vi "Error Library.vi"(0 "Path":path, 2 "action":T2=enum."Register", 7 "Priority":bool, 11 "error in":errorcluster) -> (4 "Entry":T1, 8 "found?":bool, 15 "error thru":errorcluster)   [LabVIEW 2020]
uses:
  Error-Library Action.ctl
  Error Description.ctl
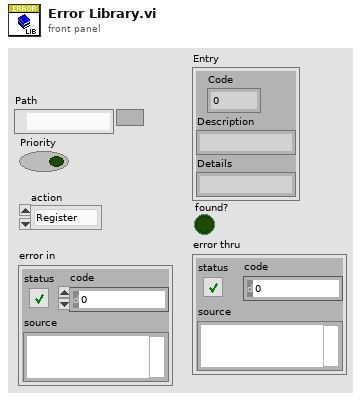
[diagram p1: front panel]
types:
  T1 = typedef "Error Description.ctl" = cluster{"Code":i32, "Description":string, "Details":string}
  T2 = typedef "Error-Library Action.ctl" = enum16{"NONE", "Register", "Read"}
  T3 = cluster{"code":i32, "source":string, "source":string}
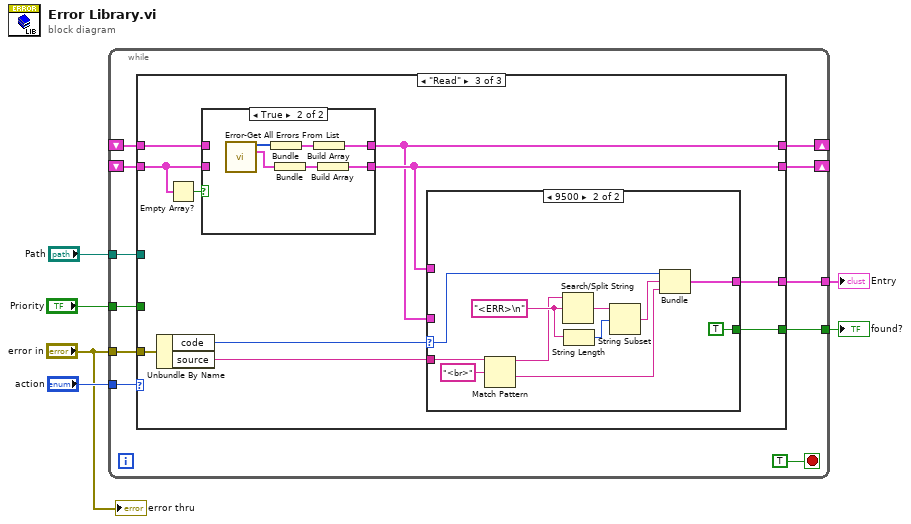
[diagram p0: block diagram]
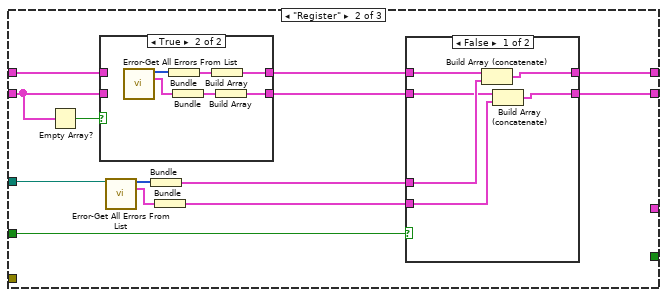
[diagram p3: hidden frame]
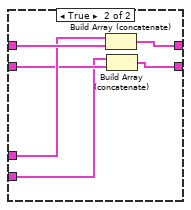
[diagram p4: hidden frame]
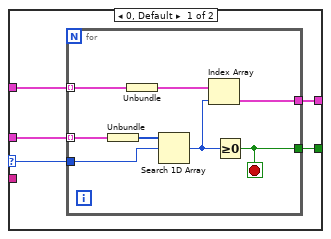
[diagram p6: hidden frame]
diagram:
  n1 = while {
    tunnel: "Path" -> [w16]
    tunnel: "Priority" -> [w15]
    tunnel: "action" -> [w14]
    shift-right: [w13] -> _
    shift-left: _ -> [w12]
    shift-right: [w11] -> _
    shift-left: _ -> [w10]
    tunnel: "error in" -> [w9]
    tunnel: [w8] -> w2
    tunnel: [w7] -> w1
    stop <- TRUE stop-if-true
    n2 = case shown="\"Read\"" w14 {
      tunnel: w16 -> [_ w27 _]
      tunnel: w15 -> [_ w22 _]
      tunnel: [w18 w23 w55] -> w13
      tunnel: w12 -> [w18 w30 w56]
      tunnel: [w19 w24 w54] -> w11
      tunnel: w10 -> [w19 w31 w57]
      tunnel: w9 -> [_ _ w62]
      tunnel: [_ _ w60] -> w8
      tunnel: [_ _ w59] -> w7
      frame "NONE", Default {
      }
      frame "Register" {
        n3 = Empty Array?(array=w30) -> (empty?=w32:bool)
        n4 = case shown="True" w32 {
          tunnel: [w46 w50] -> w26
          tunnel: [w45 w47] -> w25
          tunnel: w31 -> [w46 _]
          tunnel: w30 -> [w45 _]
          frame False {
          }
          frame True {
            n5 = call "Error-Get All Errors From List.vi"() -> ("Codes"=w52:i32[], "Errors"=w48:T1[])  [unwired: 13 in, 1 out]
            n6 = Bundle("Codes"=w52) -> (w51:cluster{"Codes":i32[]})  [unwired: 1 in]
            n7 = Bundle("Errors"=w48) -> (w49:cluster{"Errors":T1[]})  [unwired: 1 in]
            n8 = Build Array(w51) -> (w50:cluster{"Codes":i32[]}[])
            n9 = Build Array(w49) -> (w47:cluster{"Errors":T1[]}[])
          }
        }
        n10 = call "Error-Get All Errors From List.vi"("Path"=w27) -> ("Codes"=w29:i32[], "Errors"=w28:T1[])  [unwired: 12 in, 1 out]
        n11 = Bundle("Codes"=w29) -> (w21:cluster{"Codes":i32[]})  [unwired: 1 in]
        n12 = Bundle("Errors"=w28) -> (w20:cluster{"Errors":T1[]})  [unwired: 1 in]
        n13 = case shown="False" w22 {
          tunnel: w26 -> [w38 w44]
          tunnel: w25 -> [w35 w41]
          tunnel: [w36 w43] -> w24
          tunnel: [w33 w40] -> w23
          tunnel: w21 -> [w37 w42]
          tunnel: w20 -> [w34 w39]
          frame False {
            n14 = Build Array (concatenate)(w38, w37) -> (w36:cluster{"Codes":i32[]}[])
            n15 = Build Array (concatenate)(w35, w34) -> (w33:cluster{"Errors":T1[]}[])
          }
          frame True {
            n16 = Build Array (concatenate)(w42, w44) -> (w43:cluster{"Codes":i32[]}[])
            n17 = Build Array (concatenate)(w39, w41) -> (w40:cluster{"Errors":T1[]}[])
          }
        }
      }
      frame "Read" {
        n18 = Unbundle By Name(w62) -> ("code"=w61:i32, "source"=w53:string)
        n19 = Empty Array?(array=w56) -> (empty?=w58:bool)
        n20 = case shown="True" w58 {
          tunnel: [w88 w92] -> w54
          tunnel: [w87 w89] -> w55
          tunnel: w57 -> [w88 _]
          tunnel: w56 -> [w87 _]
          frame False {
          }
          frame True {
            n21 = call "Error-Get All Errors From List.vi"() -> ("Codes"=w94:i32[], "Errors"=w90:T1[])  [unwired: 13 in, 1 out]
            n22 = Bundle("Codes"=w94) -> (w93:cluster{"Codes":i32[]})  [unwired: 1 in]
            n23 = Bundle("Errors"=w90) -> (w91:cluster{"Errors":T1[]})  [unwired: 1 in]
            n24 = Build Array(w93) -> (w92:cluster{"Codes":i32[]}[])
            n25 = Build Array(w91) -> (w89:cluster{"Errors":T1[]}[])
          }
        }
        n26 = case shown="9500" w61 {
          selector: w61 -> [w67 w84]
          tunnel: [w66 w82] -> w60
          tunnel: [w65 TRUE] -> w59
          tunnel: w55 -> [w64 _]
          tunnel: w54 -> [w63 _]
          tunnel: w53 -> [_ w85]
          frame 0, Default {
            n27 = for {
              tunnel: w63 -> [w75] mode=indexing
              tunnel: w64 -> [w72] mode=indexing
              tunnel: w67 -> [w73]
              tunnel: [w69] -> w66
              tunnel: [w68] -> w65
              stop <- w68 stop-if-true
              n28 = Unbundle(w75) -> ("Codes"=w74:i32[])
              n29 = Unbundle(w72) -> ("Errors"=w71:T1[])
              n30 = Search 1D Array(1D array=w74, element=w73) -> (index of element=w70:i32)  [unwired: 1 in]
              n31 = Index Array(array=w71, index=w70) -> (element=w69:T1)
              n32 = Greater Or Equal To 0?(x=w70) -> (x >= 0?=w68:bool)
            }
          }
          frame 9500 {
            w78 = "<ERR>\n" ("search string/char (-)")
            n33 = Match Pattern(string=w85, regular expression="<br>") -> (before substring=w77:string, after substring=w83:string)  [unwired: 1 in, 2 out]
            n34 = Search/Split String(string=w77, search string/char (-)=w78) -> (match + rest of string=w80:string)  [unwired: 1 in, 2 out]
            n35 = String Length(string=w78) -> (length=w79:i32)
            n36 = String Subset(string=w80, offset (0)=w79) -> (substring=w76:string)  [unwired: 1 in]
            n37 = Bundle("code"=w84, "source"=w76, "source"=w83) -> (w82:T3)  [unwired: 1 in]
          }
        }
      }
    }
  }
  "Entry" <- w2
  "found?" <- w1
  "error thru" <- "error in"
